vi "test_TCP_TCP Read.vi"(8 "error in (no error)":errorcluster, 11 "TestCase in":refnum<class "Ethernet Protocol Tests.lvclass">) -> (0 "error out":errorcluster, 3 "TestCase out":refnum<class "Ethernet Protocol Tests.lvclass">)   [LabVIEW 2019, in "Ethernet Protocol Tests.lvclass"]
uses:
  Ethernet Protocol Tests.lvclass
  Listener/Listener.lvclass
  TCP/TCP.lvclass
  D:/GitRepository/niveristand-instrument-addon-classes/Source/Protocols/Protocol Parent/Protocol Parent.lvclass
  Listener/ListenerClassControls/Operation.ctl
  TCP/TCP.lvclass/TCP.ctl
  Protocol Parent/Methods/Read Parameter.ctl
  <vilib>/addons/_JKI Toolkits/VI Tester/TestCase.llb/TestCase.lvclass
  Protocol Parent/Protocol Parent.lvclass
  C:/Program Files (x86)/National Instruments/LabVIEW 2019/vi.lib/addons/_JKI Toolkits/VI Tester/TestCase.llb/TestCase.lvclass
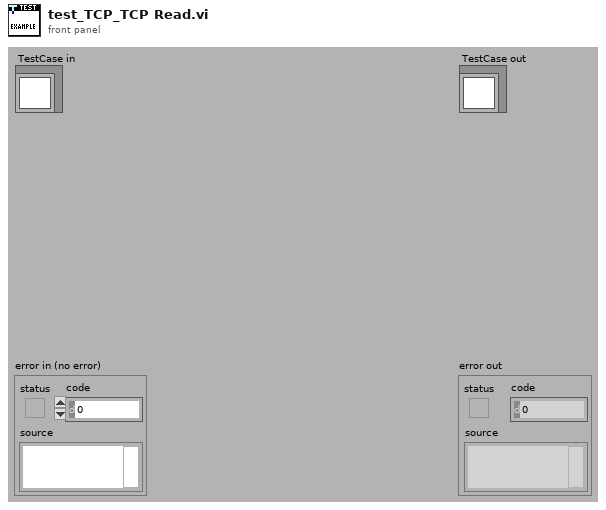
[diagram p1: front panel]
types:
  T1 = typedef "Protocols.lvlib/Protocol Parent.lvclass/Read Parameter.ctl" = cluster{"Wait Type":enum16{"Byte Count", "Wait sec"}, "Wait Value":dbl}
  T2 = typedef "Listener.lvclass/Operation.ctl" = enum16{"Read", "Write"}
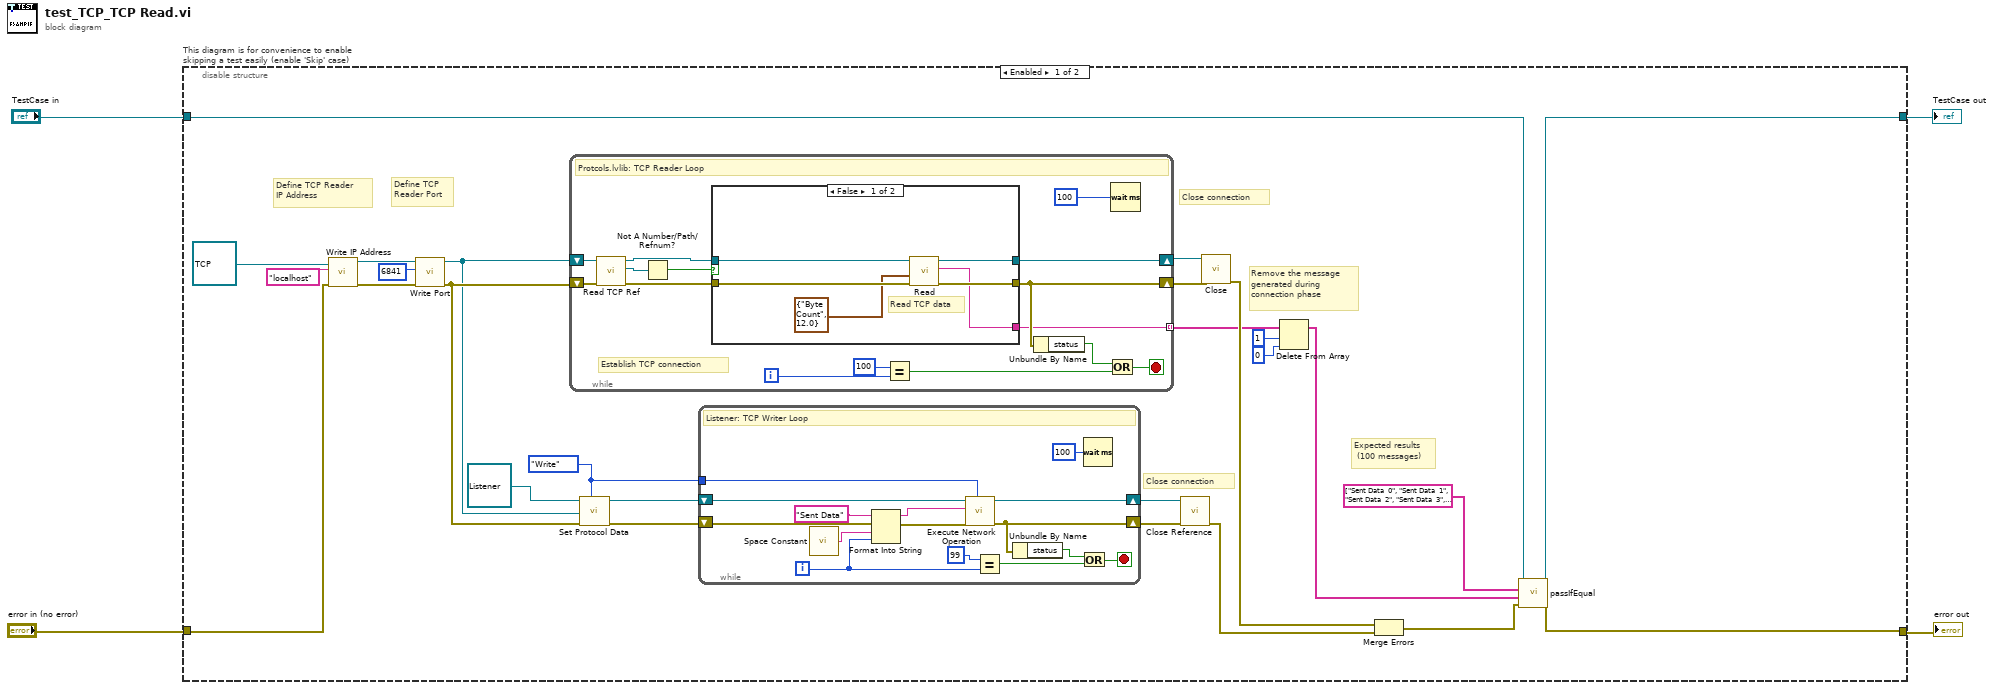
[diagram p0: block diagram]
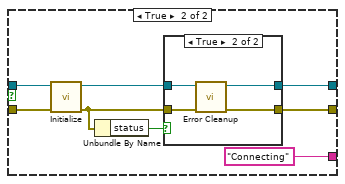
[diagram p2: hidden frame]
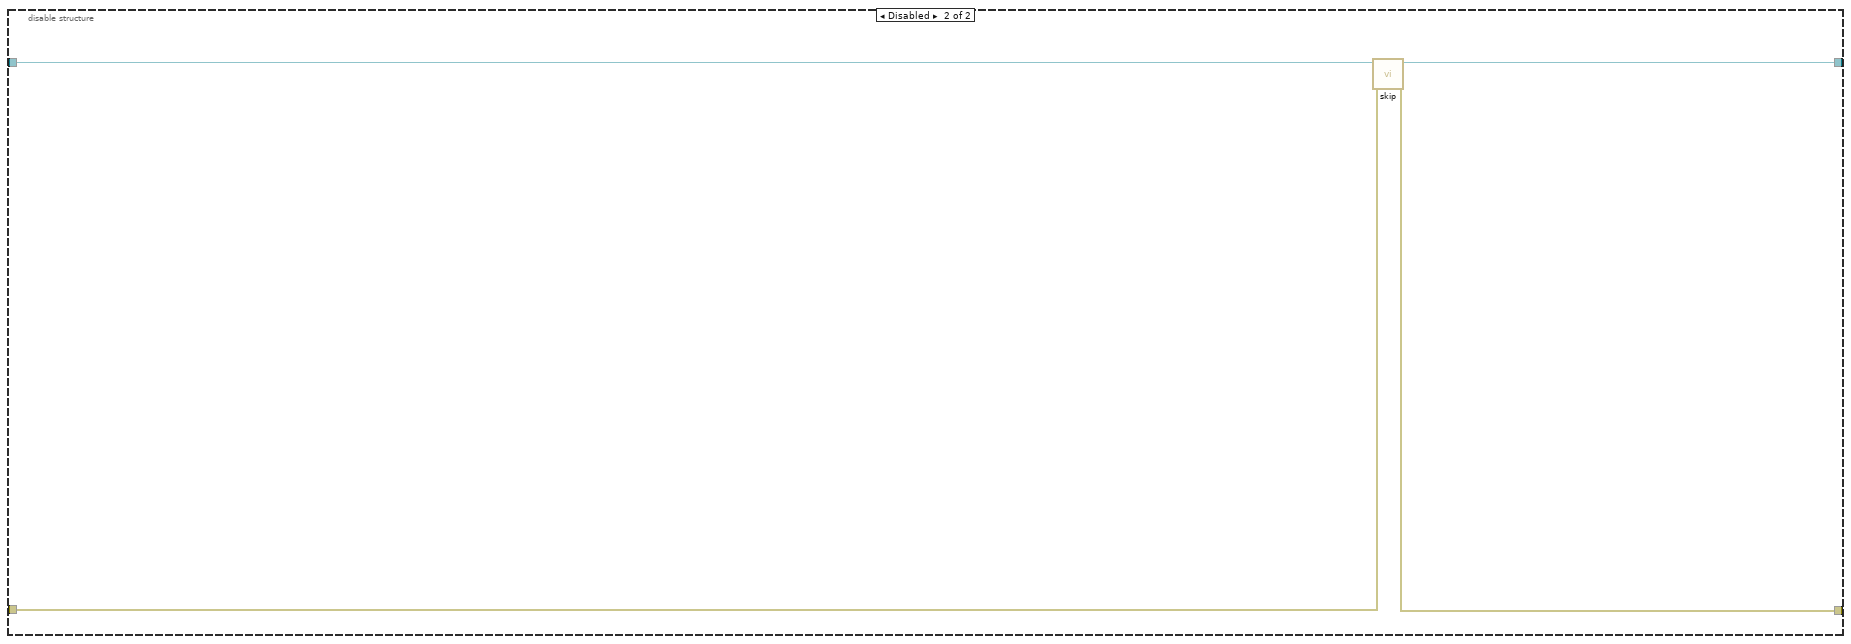
[diagram p4: hidden frame]
diagram:
  n1 = disable-structure "This diagram is for convenience to enable skipping a test easily (enable 'Skip' case)" shown="Enabled" {
    disable-tunnel: "TestCase in" -> [w31 w85]
    disable-tunnel: [w30 w83] -> w1
    disable-tunnel: [w29 w84] -> w3
    disable-tunnel: "error in (no error)" -> [w24 w82]
    frame Enabled {
      w9 = Operation."Write" ("Operation")
      # "Close connection"
      # "Close connection"
      # "Remove the message\ngenerated during \nconnection phase"
      # "Expected results\n (100 messages)"
      # "Define TCP \nReader Port"
      # "Define TCP Reader \nIP Address"
      n2 = call "Write IP Address.vi"("error in (no error)"=w24, "IP Address"="localhost", "Ethernet in"=refnum<class "TCP.lvclass"> refnum ("Protocols.lvlib:TCP.lvclass")) -> ("error out"=w26:errorcluster, "Ethernet out"=w27:refnum<class "TCP.lvclass">)  [unwired: 7 in]
      n3 = call "Write Port.vi"("error in (no error)"=w26, "Port"=u16 6841, "Ethernet in"=w27) -> ("error out"=w8:errorcluster, "Ethernet out"=w7:refnum<class "TCP.lvclass">)  [unwired: 7 in]
      n4 = while {
        shift-right: [w54] -> w19
        shift-left: w8 -> [w51]
        shift-right: [w61] -> w18
        shift-left: w7 -> [w52]
        tunnel: [w53] -> w6 mode=indexing
        i -> [w60]
        stop <- w56 stop-if-true
        # "Establish TCP connection"
        # "Protcols.lvlib: TCP Reader Loop"
        n5 = call "Read TCP Ref.vi"("error in (no error)"=w51, "Ethernet in"=w52) -> ("error out"=w47:errorcluster, "TCP Ref"=w50:refnum<k5>, "Ethernet out"=w48:refnum<class "TCP.lvclass">)  [unwired: 7 in]
        n6 = Not A Number/Path/Refnum?(number/path/refnum=w50) -> (NaN/Path/Refnum?=w49:bool)
        n7 = case shown="False" w49 {
          tunnel: w48 -> [w67 w74]
          tunnel: w47 -> [w66 w75]
          tunnel: [w65 w72] -> w61
          tunnel: [w63 w71] -> w54
          tunnel: [w62 "Connecting" ("String")] -> w53
          frame False {
            # "Read TCP data"
            n8 = call-dynamic "Read.vi"("error in (no error)"=w66, "Variant"=T1 {"Wait Type"=enum."Byte Count", "Wait Value"=12.0} ("Read Parameter"), "Ethernet in"=w67) -> ("error out"=w63:errorcluster, "String"=w62:string, "Ethernet out"=w65:refnum<class "TCP.lvclass">)  [unwired: 6 in]
          }
          frame True {
            n9 = call-dynamic "Initialize.vi"("error in (no error)"=w75, "Ethernet in"=w74) -> ("error out"=w69:errorcluster, "Ethernet out"=w73:refnum<class "TCP.lvclass">)  [unwired: 8 in]
            n10 = Unbundle By Name(w69) -> ("status"=w68:bool)
            n11 = case shown="True" w68 {
              tunnel: w69 -> [w76 w81]
              tunnel: w73 -> [w77 w80]
              tunnel: [w77 w79] -> w72
              tunnel: [w76 w78] -> w71
              frame False {
              }
              frame True {
                n12 = call-dynamic "Error Cleanup.vi"("error in (no error)"=w81, "Ethernet in"=w80) -> ("error out"=w78:errorcluster, "Ethernet out"=w79:refnum<class "TCP.lvclass">)  [unwired: 8 in]
              }
            }
          }
        }
        n13 = Equal?(x=100, y=w60) -> (x = y?=w57:bool)
        n14 = Unbundle By Name(w54) -> ("status"=w58:bool)
        n15 = Or(x=w58, y=w57) -> (x .or. y?=w56:bool)
        n16 = Wait (ms)(milliseconds to wait=u32 100) -> ()  [unwired: 1 out]
      }
      n17 = call "Set Protocol Data.vi"("Operation"=w9, "error in (no error)"=w8, "Protocols.lvlib:Protocol Parent.lvclass"=w7, "Listener In.lvclass"=refnum<class "Listener.lvclass"> refnum ("Listener.lvclass")) -> ("error out"=w11:errorcluster, "Listener Out.lvclass"=w10:refnum<class "Listener.lvclass">)  [unwired: 6 in]
      n18 = while {
        shift-right: [w42] -> w15
        shift-left: w11 -> [w33]
        shift-right: [w41] -> w16
        shift-left: w10 -> [w34]
        tunnel: w9 -> [w32]
        i -> [w37]
        stop <- w45 stop-if-true
        # "Listener: TCP Writer Loop"
        n19 = call <vilib>:"Space Constant.vi"() -> ("String"=w38:string)
        n20 = Format Into String(initial string="Sent Data", error in=w33, w38, w37) -> (resulting string=w36:string, error out=w35:errorcluster)  [unwired: 1 in]
        n21 = call "Execute Network Operation.vi"("Operation"=w32, "error in (no error)"=w35, "Message"=w36, "Listener In.lvclass"=w34) -> ("error out"=w42:errorcluster, "Listener Out.lvclass"=w41:refnum<class "Listener.lvclass">)  [unwired: 6 in]
        n22 = Equal?(x=99, y=w37) -> (x = y?=w43:bool)
        n23 = Unbundle By Name(w42) -> ("status"=w46:bool)
        n24 = Or(x=w46, y=w43) -> (x .or. y?=w45:bool)
        n25 = Wait (ms)(milliseconds to wait=u32 100) -> ()  [unwired: 1 out]
      }
      n26 = call "Close Reference.vi"("error in (no error)"=w15, "Listener In.lvclass"=w16) -> ("error out"=w14:errorcluster)  [unwired: 9 in]
      n27 = call-dynamic "Close.vi"("error in (no error)"=w19, "Ethernet in"=w18) -> ("error out"=w17:errorcluster)  [unwired: 8 in, 1 out]
      n28 = Delete From Array(array=w6, length=1 ("index"), index=0 ("length")) -> (array with subset deleted=w20:string[])  [unwired: 1 out]
      n29 = Merge Errors(w17, w14) -> (w23:errorcluster)
      n30 = call-dynamic "passIfEqual.vi"("error in (no error)"=w23, "y"=w20, "x"=string[] ["Sent Data  0", "Sent Data  1", "Sent Data  2", "Sent Data  3", "Sent Data  4", "Sent Data  5", "Sent Data  6", "Sent Data  7", "Sent Data  8", "Sent Data  9", "Sent Data  1", "0Sent Data  ", "11Sent Data ", " 12Sent Data", "  13Sent Dat", "a  14Sent Da", "ta  15Sent D", "ata  16Sent ", "Data  17Sent", " Data  18Sen", "t Data  19Se", "nt Data  20S", "ent Data  21", "Sent Data  2", "2Sent Data  ", "23Sent Data ", " 24Sent Data", "  25Sent Dat", "a  26Sent Da", "ta  27Sent D", "ata  28Sent ", "Data  29Sent", " Data  30Sen", "t Data  31Se", "nt Data  32S", "ent Data  33", "Sent Data  3", "4Sent Data  ", "35Sent Data ", " 36Sent Data", "  37Sent Dat", "a  38Sent Da", "ta  39Sent D", "ata  40Sent ", "Data  41Sent", " Data  42Sen", "t Data  43Se", "nt Data  44S", "ent Data  45", "Sent Data  4", "6Sent Data  ", "47Sent Data ", " 48Sent Data", "  49Sent Dat", "a  50Sent Da", "ta  51Sent D", "ata  52Sent ", "Data  53Sent", " Data  54Sen", "t Data  55Se", "nt Data  56S", "ent Data  57", "Sent Data  5", "8Sent Data  ", "59Sent Data ", " 60Sent Data", "  61Sent Dat", "a  62Sent Da", "ta  63Sent D", "ata  64Sent ", "Data  65Sent", " Data  66Sen", "t Data  67Se", "nt Data  68S", "ent Data  69", "Sent Data  7", "0Sent Data  ", "71Sent Data ", " 72Sent Data", "  73Sent Dat", "a  74Sent Da", "ta  75Sent D", "ata  76Sent ", "Data  77Sent", " Data  78Sen", "t Data  79Se", "nt Data  80S", "ent Data  81", "Sent Data  8", "2Sent Data  ", "83Sent Data ", " 84Sent Data", "  85Sent Dat", "a  86Sent Da", "ta  87Sent D", "ata  88Sent ", "Data  89Sent", " Data  90Sen", "t Data  91Se", "nt Data  92S"] ("array w/ subset deleted"), "TestCase in"=w31) -> ("error out"=w29:errorcluster, "TestCase out"=w30:refnum<class "Ethernet Protocol Tests.lvclass">)  [unwired: 6 in]
    }
    frame Disabled {
      # "skip test result while test is under development"
      n31 = call <vilib>:"skip.vi"("error in (no error)"=w82, "TestCase in"=w85) -> ("error out"=w84:errorcluster, "TestCase out"=w83:refnum<class "Ethernet Protocol Tests.lvclass">)  [unwired: 8 in]
    }
  }
  "error out" <- w3
  "TestCase out" <- w1
